vi "Add Scalar.vi"(5 "Action":T2, 7 "SysDef Name":string, 8 "error in (no error)":errorcluster, 10 "Register Index":i32, 11 "Node Ptr in":T1 format="%.0x") -> (0 "error out":errorcluster, 3 "Node Ptr out":T1=18446744073709551615 format="%.0x")   [LabVIEW 2018, in "Scripting API.lvlib"]
uses:
  Scripting API.lvlib
  Addon/Addon System Explorer/Types/Channel Type.ctl
  <vilib>/NI Veristand/Custom Device API/Custom Device Item Ref.ctl
  Addon/Addon Shared/Types/FG Action.ctl
  Addon/Addon Shared/SubVIs/Constants.vi
  <vilib>/NI/NI VeriStand Advanced SysDef API/SysDef API/SysDef.Property.Get.vi
  <vilib>/NI/NI VeriStand Advanced SysDef API/_SubVIs/SysDef.Property.Get.Variant.vi
  <vilib>/NI/NI VeriStand Advanced SysDef API/SysDef API/SysDef.Property.Set.vi
  <vilib>/NI/NI VeriStand Advanced SysDef API/_SubVIs/SysDef.Property.Set.Variant.vi
  Addon/Addon Shared/FPGA Addon Shared.lvlib
  Addon/Addon System Explorer/FPGA Addon System Explorer.lvlib
  <vilib>/NI Veristand/Custom Device API/Custom Device API.lvlib
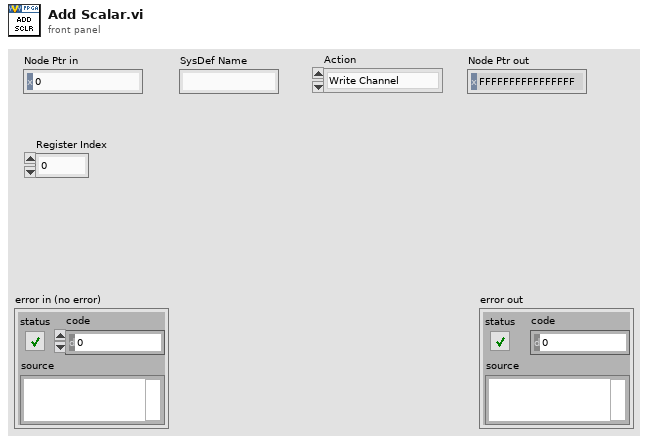
[diagram p1: front panel]
types:
  T1 = typedef "Custom Device API.lvlib/Custom Device Item Ref.ctl" = u64
  T2 = typedef "FPGA Addon System Explorer.lvlib/Channel Type.ctl" = enum16{"Write Channel", "Read Channel", "Write Waveform", "Read Waveform"}
  T3 = typedef "FPGA Addon Shared.lvlib/FG Action.ctl" = enum8{"GET", "SET"}
  T4 = typedef "FPGA Addon Shared.lvlib/Register Information.ctl" = cluster{"Name":string, "Data Type":T5, "Default Value":variant}
  T5 = typedef "FPGA Addon Shared.lvlib/Data Type.ctl" = enum8{"<Null>", "I8", "I16", "I32", "I64", "U8", "U16", "U32", "U64", "SGL", "Boolean", "Analog PWM In Settings", "Analog PWM In", "Digital PWM In Settings", "Digital PWM In", "Digital PWM Out", "Sine Out", "FXP+/-24.5", "FXP+/-16.5", "FXP+/-32.8", "FXP+/-64.32", "FXP+/-16.7", "FXP+/-20.5", "FXP+/-27.5", "FXP+/-32.16", "FXP+16.3", "FXP+18.3", "Digital Static In", "Digital Static Out", "Digital Static In Settings", "Digital WSS Out", "Quad Encoder Settings", "Quad Encoder In", "Group"}
  T6 = typedef "FPGA Addon Shared.lvlib/DMA Information.ctl" = cluster{"Name":string, "Data Type":T5}
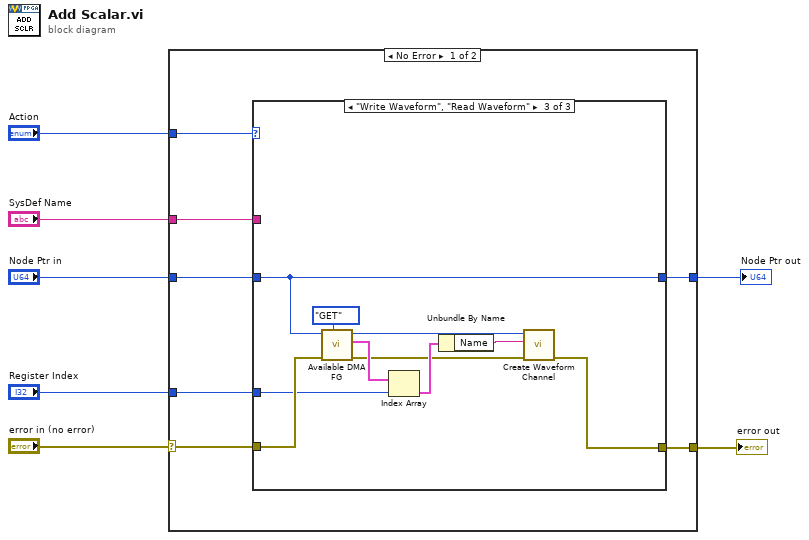
[diagram p0: block diagram]
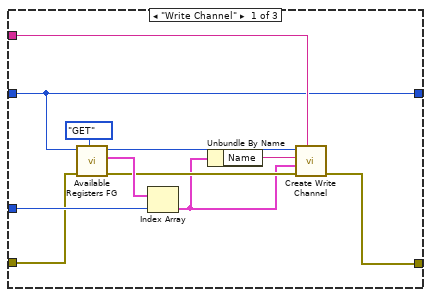
[diagram p2: hidden frame]
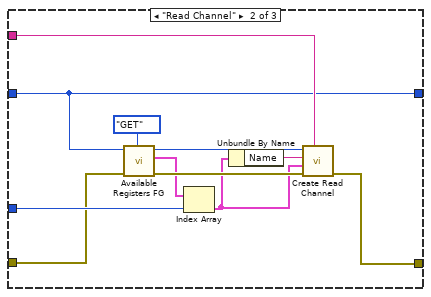
[diagram p3: hidden frame]
diagram:
  n1 = case shown="No Error" "error in (no error)" {
    selector: "error in (no error)" -> [w8 w47]
    tunnel: [w14 w47] -> w7
    tunnel: "Action" -> [w13 _]
    tunnel: "Register Index" -> [w12 _]
    tunnel: "Node Ptr in" -> [w11 w48]
    tunnel: "SysDef Name" -> [w10 _]
    tunnel: [w9 w48] -> w2
    frame No Error {
      n2 = case shown="\"Write Waveform\", \"Read Waveform\"" w13 {
        tunnel: [w21 w30 w46] -> w14
        tunnel: w11 -> [w15 w26 w38]
        tunnel: w12 -> [w22 w33 w43]
        tunnel: w8 -> [w19 w31 w45]
        tunnel: w10 -> [w18 w29 _]
        tunnel: [w15 w26 w38] -> w9
        frame "Write Channel" {
          n3 = call "Available Registers FG.vi"("Action"=FG_Action."GET", "error in (no error)"=w19, "Item Ref"=w15) -> ("error out"=w23:errorcluster, "Available Registers"=w24:T4[], "Item Ref out"=w20:T1)  [unwired: 6 in]
          n4 = Index Array(array=w24, index=w22) -> (element=w16:T4)
          n5 = Unbundle By Name(w16) -> ("Name"=w17:string)
          n6 = call "Create Write Channel.vi"("Name"=w18, "error in (no error)"=w23, "Cluster"=w16, "Bitfile Name"=w17, "Item Ref in"=w20) -> ("error out"=w21:errorcluster)  [unwired: 6 in]
        }
        frame "Read Channel" {
          n7 = call "Available Registers FG.vi"("Action"=FG_Action."GET", "error in (no error)"=w31, "Item Ref"=w26) -> ("error out"=w35:errorcluster, "Available Registers"=w34:T4[], "Item Ref out"=w32:T1)  [unwired: 6 in]
          n8 = Index Array(array=w34, index=w33) -> (element=w28:T4)
          n9 = Unbundle By Name(w28) -> ("Name"=w27:string)
          n10 = call "Create Read Channel.vi"("Name"=w29, "error in (no error)"=w35, "Channel"=w28, "Bitfile Name"=w27, "Item Ref in"=w32) -> ("error out"=w30:errorcluster)  [unwired: 6 in]
        }
        frame "Write Waveform", "Read Waveform" {
          n11 = call "Available DMA FG.vi"("Action"=FG_Action."GET", "error in (no error)"=w45, "Item Ref"=w38) -> ("error out"=w39:errorcluster, "Available DMA"=w44:T6[], "Item Ref out"=w42:T1)  [unwired: 6 in]
          n12 = Index Array(array=w44, index=w43) -> (element=w41:T6)
          n13 = Unbundle By Name(w41) -> ("Name"=w40:string)
          n14 = call "Create Waveform Channel.vi"("error in (no error)"=w39, "Bitfile Name"=w40, "Item Ref in"=w42) -> ("error out"=w46:errorcluster)  [unwired: 8 in]
        }
      }
    }
    frame Error {
    }
  }
  "error out" <- w7
  "Node Ptr out" <- w2
